vi "p1.vi"() -> ()   [LabVIEW 2023, in "d13.lvlib"]
uses:
  d13.lvlib
  0444afec-930e-4102-924f-d7b56dd744f8.vi
  298415db-d03c-438a-94ab-1c1eb124d9ea.vi
  AOC/AOC.lvlib
panel:
  in  "Example":string="#.##..##.\n..#.##.#.\n##......#\n##......#\n..#.##.#.\n..##..##.\n#.#.##.#.\n\n#...##..#\n#....#..#\n..##..###\n#####.##.\n#####.##.\n..##..###\n#....#..#"
  in  "Example":bool=TRUE
  out "Answer":u64=5675
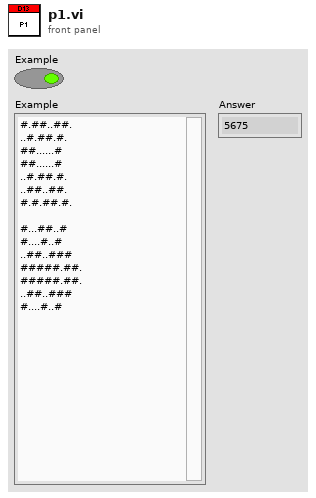
[diagram p1: front panel]
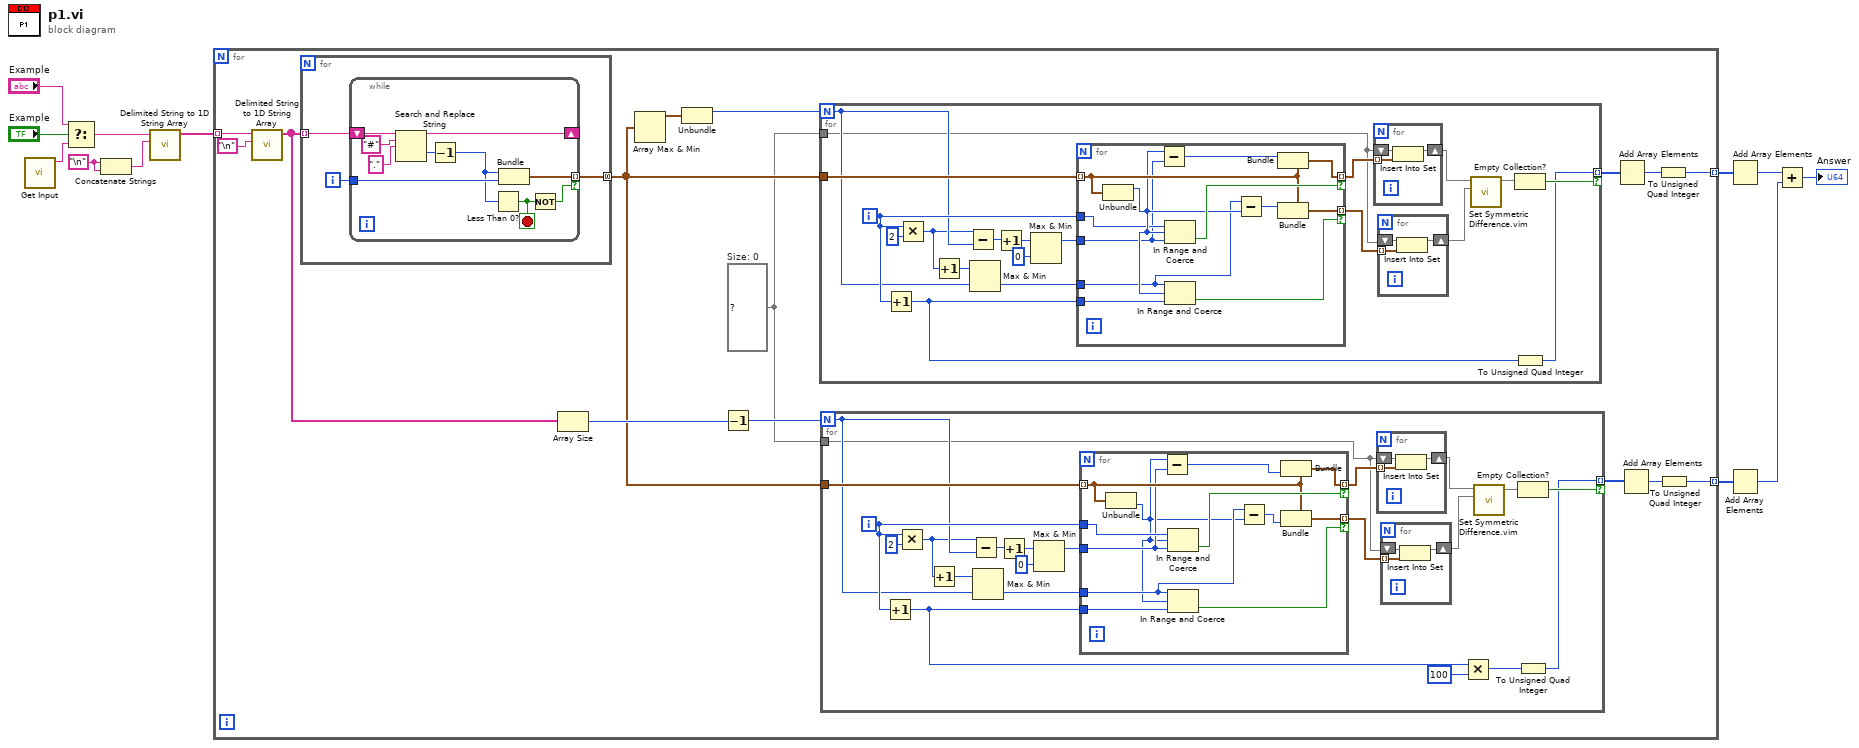
[diagram p0: block diagram]
diagram:
  w5 = "\n"
  n1 = call "Get Input.vi"() -> ("Input"=w12:string)  [unwired: 11 in]
  n2 = Select(t="Example", s="Example", f=w12) -> (s? t:f=w8:string)
  n3 = Concatenate Strings(w5, w5) -> (w6:string)
  n4 = call <vilib>:"Delimited String to 1D String Array.vi"("delimiter"=w6, "delimited string"=w8) -> ("string array"=w7:string[])  [unwired: 9 in]
  n5 = for {
    tunnel: w7 -> [w27] mode=indexing
    tunnel: [w18] -> w9 mode=indexing
    tunnel: [w21] -> w4 mode=indexing
    w13 = set{cluster{"offset of match":i32, i32}} {}  # Size: 0
    n6 = call <vilib>:"Delimited String to 1D String Array.vi"("delimiter"="\n", "delimited string"=w27) -> ("string array"=w25:string[])  [unwired: 9 in]
    n7 = for {
      tunnel: w25 -> [w68] mode=indexing
      tunnel: [w67] -> w16 mode=concatenating
      i -> [w66]
      n8 = while {
        tunnel: [w78] -> w67 mode=indexing if=w75
        tunnel: w66 -> [w77]
        shift-right: [w73] -> _
        shift-left: w68 -> [w74]
        stop <- w76 stop-if-true
        n9 = Search and Replace String(input string=w74, search string="#" ("search string/char (-)"), replace string="." ("replace string (\"\")")) -> (result string=w73:string, offset past replacement=w71:i32)  [unwired: 5 in, 2 out]
        n10 = Decrement(x=w71) -> (x-1=w70:i32)
        n11 = Less Than 0?(x=w70) -> (x < 0?=w76:bool)
        n12 = Bundle(w70, w77) -> (w78:cluster{i32, i32})  [unwired: 1 in]
        n13 = Not(x=w76) -> (.not. x?=w75:bool)
      }
    }
    n14 = Array Size(array=w25) -> (size(s)=w17:i32)
    n15 = Array Max & Min(array=w16) -> (max value=w24:cluster{i32, i32})  [unwired: 3 out]
    n16 = Unbundle(w24) -> (w23:i32)  [unwired: 1 out]
    n17 = Decrement(x=w17) -> (x-1=w14:i32)
    n18 = for {
      N: w23 -> [w37]
      tunnel: w16 -> [w47]
      tunnel: [w45] -> w20 mode=indexing if=w46
      tunnel: w13 -> [w31]
      i -> [w38]
      n19 = Increment(x=w38) -> (x+1=w32:i32)
      n20 = Multiply(x=w38, y=2) -> (x*y=w36:i32)
      n21 = Increment(x=w36) -> (x+1=w33:i32)
      n22 = Subtract(x=w36, y=w37) -> (x-y=w41:i32)
      n23 = Max & Min(x=w33, y=w37) -> (min(x,y)=w35:i32)  [unwired: 1 out]
      n24 = Increment(x=w41) -> (x+1=w40:i32)
      n25 = Max & Min(x=w40, y=0) -> (max(x,y)=w39:i32)  [unwired: 1 out]
      n26 = for {
        tunnel: w47 -> [w61] mode=indexing
        tunnel: [w60] -> w44 mode=indexing if=w63
        tunnel: [w65] -> w34 mode=indexing if=w64
        tunnel: w39 -> [w56]
        tunnel: w38 -> [w57]
        tunnel: w32 -> [w55]
        tunnel: w35 -> [w54]
        n27 = Unbundle(w61) -> (w59:i32)  [unwired: 1 out]
        n28 = Subtract(x=w59, y=w56) -> (x-y=w58:i32)
        n29 = In Range and Coerce(upper limit=w57, x=w59, lower limit=w56) -> (In Range?=w63:bool)  [unwired: 1 out]
        n30 = In Range and Coerce(upper limit=w54, x=w59, lower limit=w55) -> (In Range?=w64:bool)  [unwired: 1 out]
        n31 = Subtract(x=w54, y=w59) -> (x-y=w62:i32)
        n32 = Bundle(cluster=w61, w58) -> (w60:cluster{i32, i32})  [unwired: 1 in]
        n33 = Bundle(cluster=w61, w62) -> (w65:cluster{i32, i32})  [unwired: 1 in]
      }
      n34 = for {
        tunnel: w44 -> [w50] mode=indexing
        shift-right: [w48] -> w30
        shift-left: w31 -> [w49]
        n35 = Insert Into Set(10:w50, 11:w49) -> (3:w48:set{cluster{"offset of match":i32, i32}})  [unwired: 1 out]
      }
      n36 = for {
        tunnel: w34 -> [w53] mode=indexing
        shift-right: [w51] -> w29
        shift-left: w31 -> [w52]
        n37 = Insert Into Set(10:w53, 11:w52) -> (3:w51:set{cluster{"offset of match":i32, i32}})  [unwired: 1 out]
      }
      n38 = call "Set Symmetric Difference.vim"("set 2"=w29, "set 1"=w30) -> ("symmetric difference"=w28:set{cluster{"offset of match":i32, i32}})  [unwired: 9 in]
      n39 = Empty Collection?(1:w28) -> (0:w46:bool)
      n40 = To Unsigned Quad Integer(1:w32) -> (0:w45:u64)
    }
    n41 = for {
      N: w14 -> [w87]
      tunnel: w16 -> [w100]
      tunnel: [w95] -> w15 mode=indexing if=w96
      tunnel: w13 -> [w79]
      i -> [w88]
      n42 = Increment(x=w88) -> (x+1=w80:i32)
      n43 = Multiply(x=w88, y=2) -> (x*y=w86:i32)
      n44 = Increment(x=w86) -> (x+1=w83:i32)
      n45 = Subtract(x=w86, y=w87) -> (x-y=w91:i32)
      n46 = Max & Min(x=w83, y=w87) -> (min(x,y)=w85:i32)  [unwired: 1 out]
      n47 = Increment(x=w91) -> (x+1=w90:i32)
      n48 = Max & Min(x=w90, y=0) -> (max(x,y)=w89:i32)  [unwired: 1 out]
      n49 = for {
        tunnel: w100 -> [w115] mode=indexing
        tunnel: [w114] -> w94 mode=indexing if=w116
        tunnel: [w118] -> w84 mode=indexing if=w117
        tunnel: w89 -> [w112]
        tunnel: w88 -> [w113]
        tunnel: w80 -> [w111]
        tunnel: w85 -> [w110]
        n50 = Unbundle(w115) -> (w107:i32)  [unwired: 1 out]
        n51 = Subtract(x=w107, y=w112) -> (x-y=w109:i32)
        n52 = In Range and Coerce(upper limit=w113, x=w107, lower limit=w112) -> (In Range?=w116:bool)  [unwired: 1 out]
        n53 = In Range and Coerce(upper limit=w110, x=w107, lower limit=w111) -> (In Range?=w117:bool)  [unwired: 1 out]
        n54 = Subtract(x=w110, y=w107) -> (x-y=w108:i32)
        n55 = Bundle(cluster=w115, w109) -> (w114:cluster{i32, i32})  [unwired: 1 in]
        n56 = Bundle(cluster=w115, w108) -> (w118:cluster{i32, i32})  [unwired: 1 in]
      }
      n57 = for {
        tunnel: w94 -> [w102] mode=indexing
        shift-right: [w101] -> w98
        shift-left: w79 -> [w103]
        n58 = Insert Into Set(10:w102, 11:w103) -> (3:w101:set{cluster{"offset of match":i32, i32}})  [unwired: 1 out]
      }
      n59 = for {
        tunnel: w84 -> [w105] mode=indexing
        shift-right: [w104] -> w99
        shift-left: w79 -> [w106]
        n60 = Insert Into Set(10:w105, 11:w106) -> (3:w104:set{cluster{"offset of match":i32, i32}})  [unwired: 1 out]
      }
      n61 = Multiply(x=w80, y=100) -> (x*y=w82:i32)
      n62 = call "Set Symmetric Difference.vim"("set 2"=w99, "set 1"=w98) -> ("symmetric difference"=w97:set{cluster{"offset of match":i32, i32}})  [unwired: 9 in]
      n63 = Empty Collection?(1:w97) -> (0:w96:bool)
      n64 = To Unsigned Quad Integer(1:w82) -> (0:w95:u64)
    }
    n65 = Add Array Elements(numeric array=w20) -> (sum=w19:u64)
    n66 = Add Array Elements(numeric array=w15) -> (sum=w22:u64)
    n67 = To Unsigned Quad Integer(1:w19) -> (0:w18:u64)
    n68 = To Unsigned Quad Integer(1:w22) -> (0:w21:u64)
  }
  n69 = Add Array Elements(numeric array=w9) -> (sum=w2:u64)
  n70 = Add Array Elements(numeric array=w4) -> (sum=w3:u64)
  n71 = Add(x=w2, y=w3) -> (x+y=→"Answer":u64)
